vi "Get Plugin Summary Info.vi"(8 "error in (no error)":errorcluster, 11 "CIF_UI in":refnum<class "CIF_UI.lvclass">) -> (0 "error out":errorcluster, 1 "Plugin Summary Info":T1[](array[typedef]), 3 "CIF_UI out":refnum<class "CIF_UI.lvclass">)   [LabVIEW 2021, in "CIF_UI.lvclass"]
uses:
  CIF_UI.lvclass
  CIF_UI.lvclass/CIF_UI.ctl
  Typedef/Plugin Summary.ctl
  3cb97bbe-ec67-4187-806b-96be001ee38f.vi
  Typedef/Version.ctl
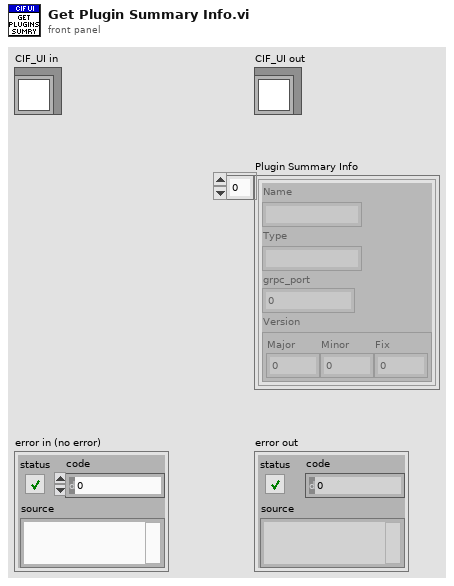
[diagram p1: front panel]
types:
  T1 = typedef "CIF_UI.lvclass/Plugin Summary.ctl" = cluster{"Name":string, "Type":string, "grpc_port":i32, "Version":T2}
  T2 = typedef "CIF_UI.lvclass/Version.ctl" = cluster{"Major":i32, "Minor":i32, "Fix":i32}
  T3 = typedef "CIF_UI.lvclass/Plugin Connection Map.ctl" = map{string, T4}
  T4 = typedef "CIF_UI.lvclass/Plugin Connections.ctl" = cluster{"gRPC ID":T5, "Plugin Info":T6}
  T5 = typedef "grpc-lvsupport-release.lvlib/grpcId.ctl" = u64
  T6 = typedef "CIF_UI.lvclass/PluginInfo.ctl" = cluster{"Name":string, "Type":string, "grpc_port":i32, "Version":T2, "Node Status":T7}
  T7 = typedef "CIFCoreCommon.lvlib/gRPC Reported Plugin Status.ctl" = cluster{"State":T8, "Timing Statistics (us)":T9, "FIFO Statistics (us)":T11, "error":T12, "Monitor Doubles":T13, "Monitor U64":T14, "Monitor I64":T15}
  T8 = typedef "CIFCoreCommon.lvlib/Plugin State.ctl" = enum32{"Null", "Creating", "Listening", "Running", "CleaningUp", "Destroying"}
  T9 = typedef "CIFCoreCommon.lvlib/Timing Statistics.ctl" = cluster{"Period":T10, "Wake Error":T10, "Execute":T10, "Housekeep":T10, "Idle":T10, "Cleanup":T10, "Custom 1 (custom units)":T10, "Custom 2 (custom units)":T10}
  T10 = typedef "CIFCoreCommon.lvlib/Timing Stats Base.ctl" = cluster{"Max":i64, "Avg":dbl, "Min":i64}
  T11 = typedef "CIFCoreCommon.lvlib/FIFO Statistics.ctl" = cluster{"From T0":T10, "From Previous Plugin":T10, "Output Error":T10}
  T12 = typedef "CIFCoreCommon.lvlib/Simple Error.ctl" = cluster{"status":bool, "code":i32}
  T13 = typedef "CIFCoreCommon.lvlib/Monitor Doubles.ctl" = cluster{"1":dbl, "2":dbl, "3":dbl, "4":dbl}
  T14 = typedef "CIFCoreCommon.lvlib/Monitor U64.ctl" = cluster{"1":u64, "2":u64, "3":u64, "4":u64}
  T15 = typedef "CIFCoreCommon.lvlib/Monitor I64.ctl" = cluster{"1":i64, "2":i64, "3":i64, "4":i64}
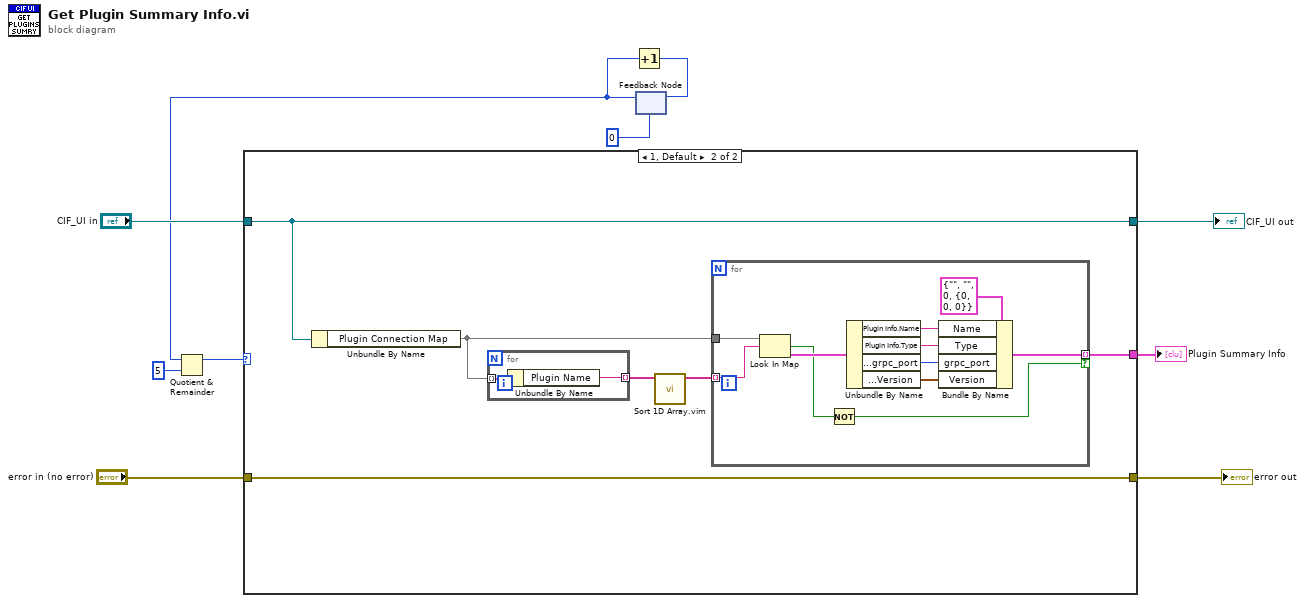
[diagram p0: block diagram]
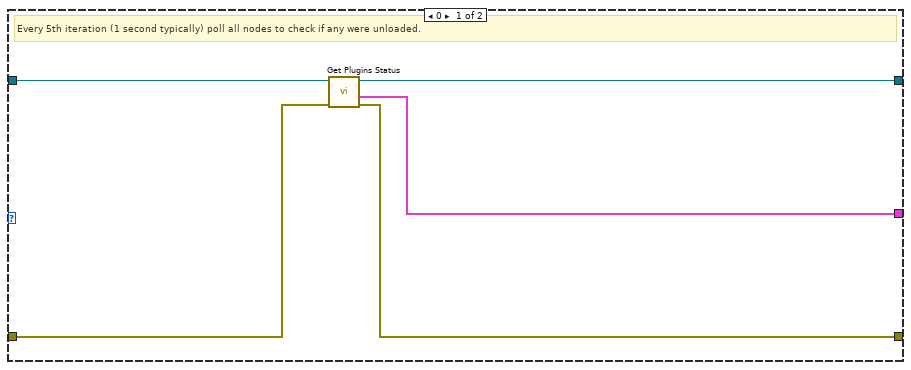
[diagram p2: hidden frame]
diagram:
  n1 = feedback #1(0) -> (w3:i32)
  n2 = Quotient & Remainder(x=w3, y=5) -> (x-y*floor(x/y)=w4:i32)  [unwired: 1 out]
  n3 = case shown="1, Default" w4 {
    tunnel: [w11 w21] -> w10
    tunnel: "CIF_UI in" -> [w15 w17]
    tunnel: [w14 w17] -> w7
    tunnel: [w12 w16] -> w6
    tunnel: "error in (no error)" -> [w13 w16]
    frame 0 {
      # "Every 5th iteration (1 second typically) poll all nodes to check if any were unloaded."
      n4 = call "Get Plugins Status.vi"("error in (no error)"=w13, "CIF_UI in"=w15) -> ("error out"=w12:errorcluster, "Plugin Summary Info"=w11:T1[], "CIF_UI out"=w14:refnum<class "CIF_UI.lvclass">)  [unwired: 6 in, 1 out]
    }
    frame 1, Default {
      n5 = Unbundle By Name(w17) -> ("Plugin Connection Map"=w18:T3)
      n6 = for {
        tunnel: w18 -> [w34] mode=indexing
        tunnel: [w33] -> w20 mode=indexing
        n7 = Unbundle By Name(w34) -> ("Plugin Name"=w33:string)
      }
      n8 = call "Sort 1D Array.vim"("unsorted array"=w20) -> ("sorted array"=w19:string[])  [unwired: 10 in]
      n9 = for {
        tunnel: [w32] -> w21 mode=indexing if=w31
        tunnel: w19 -> [w25] mode=indexing
        tunnel: w18 -> [w22]
        n10 = Look In Map(map=w22, key=w25) -> (key not found?=w23:bool, value=w24:T4)  [unwired: 1 in]
        n11 = Not(x=w23) -> (.not. x?=w31:bool)
        n12 = Unbundle By Name(w24) -> ("Plugin Info.Name"=w29:string, "Plugin Info.Type"=w26:string, "Plugin Info.grpc_port"=w27:i32, "Plugin Info.Version"=w28:T2)
        n13 = Bundle By Name(cluster=T1 {"Name"="", "Type"="", "grpc_port"=0, "Version"={"Major"=0, "Minor"=0, "Fix"=0}} ("Plugin Summary"), "Name"=w29, "Type"=w26, "grpc_port"=w27, "Version"=w28) -> (w32:T1)
      }
    }
  }
  "error out" <- w6
  "Plugin Summary Info" <- w10
  "CIF_UI out" <- w7
  n14 = Increment(x=w3) -> (x+1=w2:i32)
  n15 = feedback-in #1(w2) -> ()
